vi "Actor Core.vi"(8 "error in":errorcluster, 11 "Display Console in":refnum<class "Sensor Interface.lvclass">) -> (0 "error out":errorcluster, 3 "Actor out":refnum<class "Actor.lvclass">)   [LabVIEW 2019, in "Sensor Interface Actor.lvlib" / "Sensor Interface.lvclass"]
doc: "(<B>Filename</B>: Actor Framework.lvlib:Actor.lvclass:Actor Core.vi)\n\nReceives messages to the actor, reacts to them, and initiates any error handling that may shut the actor down.\n\nDescendant classes may override this VI to append parallel tasks for the actor to complete while it handles messages. Overrides use the Call Parent Method node."
uses:
  Sensor Interface.lvclass
  <vilib>/ActorFramework/Stop Msg/Stop Msg.lvclass
  <vilib>/ActorFramework/Actor/Actor.lvclass
  Abstract Sensor Interface Actor/Abstract Sensor Interface/Abstract Sensor Interface.lvclass
  Abstract User Console Actor/Abstract User Console Messages/Enable Door Msg/Enable Door Msg.lvclass
  C:/Workspace/CLA/Elevator AF/Abstract Sensor Interface Actor/Abstract Sensor Interface/Abstract Sensor Interface.lvclass
  C:/Program Files (x86)/National Instruments/LabVIEW 2019/vi.lib/ActorFramework/Actor/Actor.lvclass
  Elevator Position.ctl
panel:
  in  "Elevator Position":T1 scale=1.0..4.0
  # "[Covers: UI1]"
  # "[Covers: UI4] \n[Covers: UI4A]"
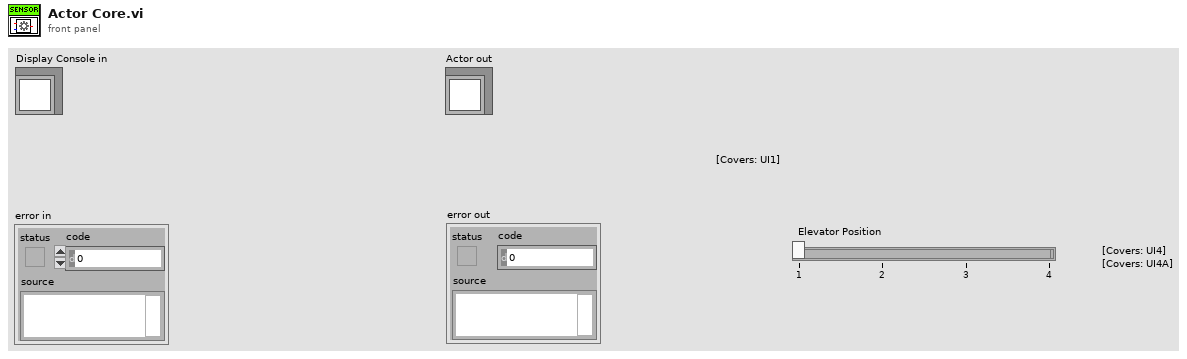
[diagram p1: front panel]
types:
  T1 = typedef "Sensor Interface Actor.lvlib/Sensor Interface.lvclass/Elevator Position.ctl" = u8
  T2 = enum8{"Enabled", "Disabled", "Disabled and Grayed Out"}
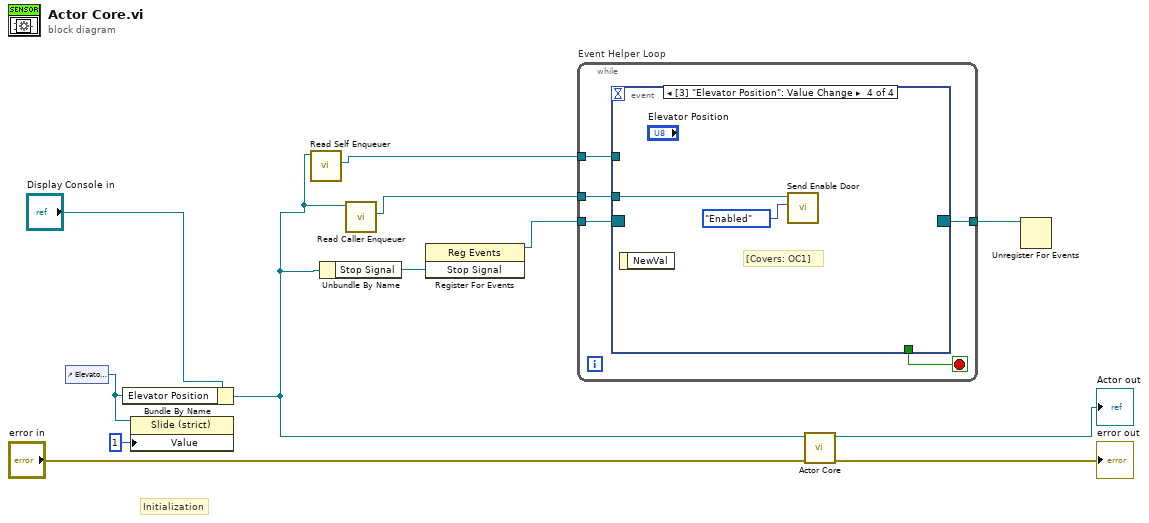
[diagram p0: block diagram]
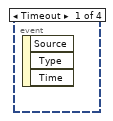
[diagram p2: hidden frame]
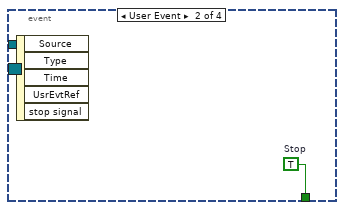
[diagram p3: hidden frame]
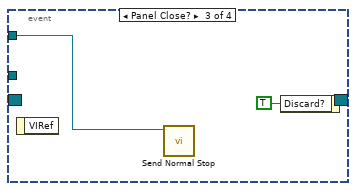
[diagram p4: hidden frame]
diagram:
  # "Initialization"
  n1 = control-ref of="Elevator Position"() -> (w4:refnum<vi>)
  n2 = Bundle By Name(cluster="Display Console in", "Elevator Position"=w4) -> (w2:refnum<class "Sensor Interface.lvclass">)
  n3 = property class="Slide (strict)"(reference=w4, "Value"=u8 1) -> ()  [unwired: 1 in, 2 out]
  n4 = call <vilib>:"Read Self Enqueuer.vi"("Actor"=w2) -> ("Self Enqueuer"=w6:refnum<class "Message Enqueuer.lvclass">)  [unwired: 10 in]
  n5 = Unbundle By Name(w2) -> ("Stop Signal"=w9:refnum<user-event>)
  n6 = call <vilib>:"Read Caller Enqueuer.vi"("Actor"=w2) -> ("Caller Enqueuer"=w1:refnum<class "Message Enqueuer.lvclass">)  [unwired: 10 in]
  n7 = register-events(w9) -> (reference out=w8:refnum<event-registration>)  [unwired: 2 in, 1 out]
  n8 = while "Event Helper Loop" {
    tunnel: w6 -> [w17]
    tunnel: w8 -> [w16]
    tunnel: [w15] -> w7
    tunnel: w1 -> [w13]
    stop <- w14 stop-if-true
    n9 = event shown="[3] \"Elevator Position\": Value Change" {
      selector: w16 -> [_ _ _ _]
      dyn-events: [_ _ _ _] -> w15
      timeout: _ -> [_ _ _ _]
      tunnel: w17 -> [_ _ w20 _]
      tunnel: [_ w18 _ _] -> w14
      tunnel: w13 -> [_ _ _ w22]
      event Timeout {
        n10 = event-data() -> ()  [unwired: 1 in, 3 out]
      }
      event User Event {
        w18 = TRUE  # Stop
        n11 = event-data() -> ()  [unwired: 1 in, 5 out]
      }
      event Panel Close? {
        n12 = event-data() -> ()  [unwired: 1 in, 1 out]
        n13 = call <vilib>:"Send Normal Stop.vi"("Message Enqueuer"=w20) -> ()  [unwired: 10 in, 1 out]
        n14 = event-data("Discard?"=TRUE) -> ()  [unwired: 1 in, 1 out]
      }
      event Value Change {
        # "[Covers: OC1]"
        n15 = event-data() -> ()  [unwired: 1 in, 1 out]
        n16 = call "Send Enable Door.vi"("Disabled"=T2."Enabled", "Message Enqueuer"=w22) -> ()  [unwired: 8 in, 2 out]
      }
    }
  }
  n17 = call-parent "Actor Core.vi"("error in"="error in", "Actor in"=w2) -> ("error out"=→"error out":errorcluster, "Actor out"=→"Actor out":refnum<class "Actor.lvclass">)  [unwired: 8 in]
  n18 = Unregister For Events(event registration refnum=w7) -> ()  [unwired: 1 in, 1 out]
